vi "FFT Power Spectral Density for 1 Chan.vi"(6 "averaging parameters":T1={"averaging mode"=enum."No averaging", "weighting mode"=enum."Exponential", "number of averages"=10} {"number of averages" min=1}, 7 "restart averaging (F)":bool, 8 "error in (no error)":errorcluster, 9 "dB On (F)":bool, 10 "window":T2=1 items=["Rectangle"=0, "Hanning"=1, "Hamming"=2, "Blackman-Harris"=3, "Exact Blackman"=4, "Blackman"=5, "Flat Top"=6, "4 Term B-Harris "=7, "7 Term B-Harris"=8, "Low Sidelobe"=9, "Blackman Nuttall"=11, "Triangle"=30, "Bartlett-Hanning"=31, "Bohman"=32, "Parzen"=33, "Welch"=34, "Kaiser"=60, "Dolph-Chebyshev"=61, "Gaussian"=62], 11 "time signal":waveform(dbl)) -> (0 "error out":errorcluster, 1 "averages completed":dbl, 3 "power spectral density":cluster{"f0":dbl, "df":dbl, "magnitude":dbl[]} {"magnitude" format="%.2p"; "f0" format="%0.2p"; "df" format="%0.2p"}, 5 "averaging done":bool)   [LabVIEW 2020, in "NI_MAPro.lvlib"]
doc: "Computes the averaged power spectral density of <B>time signal</B>. The data type you wire to the <B>time signal</B> input determines the polymorphic instance to use."
uses:
  NI_MAPro.lvlib
  windowTd.ctl
  NI_AALPro.lvlib
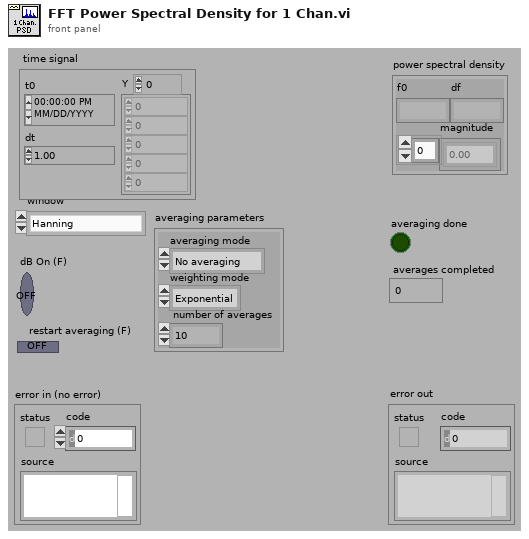
[diagram p1: front panel]
types:
  T1 = cluster{"averaging mode":enum16{"No averaging", "Vector averaging", "RMS averaging", "Peak hold"}, "weighting mode":enum16{"Linear", "Exponential"}, "number of averages":u32}
  T2 = typedef "NI_AALPro.lvlib/windowTd.ctl" = u32
  T3 = cluster{"block size":i32, "dt":dbl, "spectrum parameters":cluster{"averaging parameters":cluster{"averaging mode":enum16{"No averaging", "Vector averaging", "RMS averaging", "Peak hold"}, "weighting mode":enum16{"Linear", "Exponential"}, "number of averages":u32}, "window":T2}, "df":dbl, "averages completed":dbl, "complex spectrum":cdb[], "real spectrum":dbl[], "t0 history":dbl, "dt history":dbl, "timestamp":dbl, "lin avg done":bool}
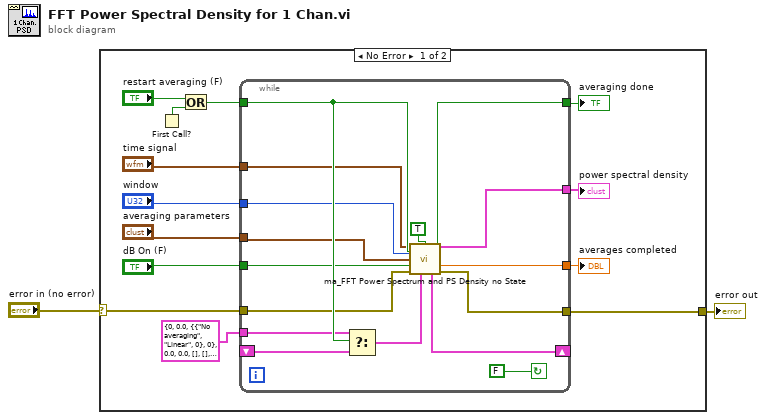
[diagram p0: block diagram]
diagram:
  n1 = case shown="No Error" "error in (no error)" {
    selector: "error in (no error)" -> [w4 w32]
    tunnel: [w8 w32] -> w2
    frame No Error {
      n2 = First Call?() -> (First Call?: T/F=w15:bool)
      n3 = Or(x="restart averaging (F)", y=w15) -> (x .or. y?=w13:bool)
      n4 = while {
        tunnel: "window" -> [w22]
        tunnel: w4 -> [w24]
        tunnel: "time signal" -> [w21]
        tunnel: "averaging parameters" -> [w20]
        tunnel: w13 -> [w26]
        tunnel: [w31] -> w5
        tunnel: [w30] -> w7
        tunnel: [w29] -> w6
        tunnel: [w28] -> w8
        shift-right: [w27] -> _
        shift-left: _ -> [w17]
        tunnel: T3 {"block size"=0, "dt"=0.0, "spectrum parameters"={"averaging parameters"={"averaging mode"=enum."No averaging", "weighting mode"=enum."Linear", "number of averages"=0}, "window"=0}, "df"=0.0, "averages completed"=0.0, "complex spectrum"=[], "real spectrum"=[], "t0 history"=0.0, "dt history"=0.0, "timestamp"=0.0, "lin avg done"=FALSE} ("state info") -> [w25]
        tunnel: "dB On (F)" -> [w23]
        stop <- FALSE continue-if-true
        n5 = Select(t=w25, s=w26, f=w17) -> (s? t:f=w18:T3)
        n6 = call "ma_FFT Power Spectrum and PS Density no State.vi"("time signal"=w21, "restart averaging (F)"=w26, "ps density"=TRUE, "window"=w22, "averaging parameters"=w20, "dB On (F)"=w23, "error in"=w24, "state info"=w18) -> ("averaging done"=w31:bool, "power spectrum"=w29:cluster{"f0":dbl, "df":dbl, "magnitude":dbl[]}, "averages completed"=w30:dbl, "state info"=w27:T3, "error out"=w28:errorcluster)  [unwired: 1 in, 2 out]
      }
      "averaging done" <- w5
      "averages completed" <- w7
      "power spectral density" <- w6
    }
    frame Error {
    }
  }
  "error out" <- w2
